vi "Send Read Geo Coding Results.vi"(7 "Message Priority (Normal)":T2=enum."Normal", 8 "error in (no error)":errorcluster, 10 "Geo Code Results":T1(array[cluster]), 11 "Message Enqueuer":refnum<class "Message Enqueuer.lvclass">) -> (0 "error out":errorcluster, 3 "Message Enqueuer out":refnum<class "Message Enqueuer.lvclass">)   [LabVIEW 2025, in "UI.lvlib" / "Read Geo Coding Results Msg.lvclass"]
doc: "This VI sends the message to an actor."
uses:
  Read Geo Coding Results Msg.lvclass
  <vilib>/ActorFramework/Message Enqueuer/Message Enqueuer.lvclass
  <vilib>/ActorFramework/Message Enqueuer/Message Priority.ctl
  C:/Program Files (x86)/National Instruments/LabVIEW 2025/vi.lib/ActorFramework/Message/Message.lvclass
  Read Geo Coding Results Msg.lvclass/Read Geo Coding Results Msg.ctl
  <vilib>/ActorFramework/Message Enqueuer/Message Enqueuer.lvclass/Message Enqueuer.ctl
  <vilib>/ActorFramework/Message Priority Queue/Priority Enqueue.vi
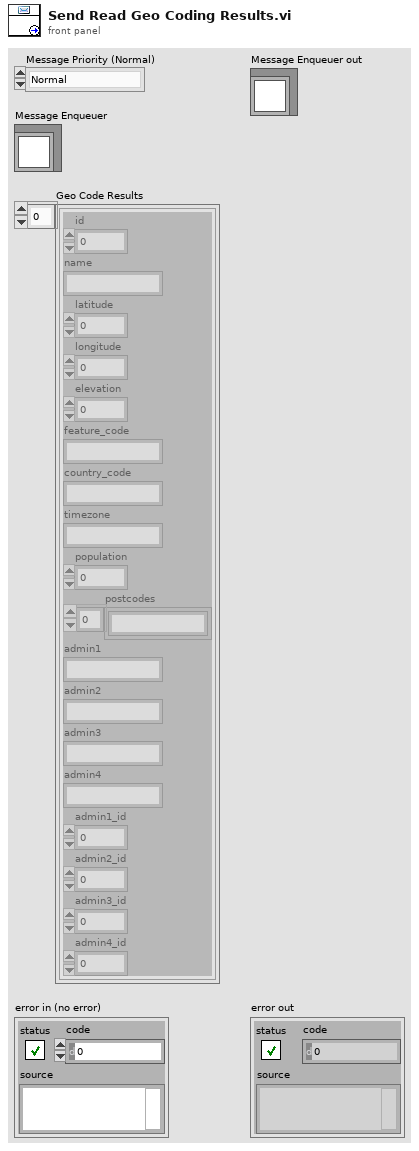
[diagram p1: front panel]
types:
  T1 = cluster{"id":i32, "name":string, "latitude":dbl, "longitude":dbl, "elevation":dbl, "feature_code":string, "country_code":string, "timezone":string, "population":i32, "postcodes":string[], "admin1":string, "admin2":string, "admin3":string, "admin4":string, "admin1_id":i32, "admin2_id":i32, "admin3_id":i32, "admin4_id":i32}[]
  T2 = typedef "Actor Framework.lvlib/Message Enqueuer.lvclass/Message Priority.ctl" = enum16{"Low", "Normal", "High"}
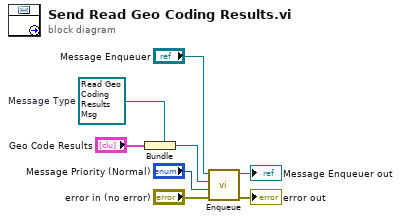
[diagram p0: block diagram]
diagram:
  w2 = refnum<class "Read Geo Coding Results Msg.lvclass"> refnum  # Message Type
  n1 = Bundle(cluster=w2, "Geo Code Results") -> (w3:refnum<class "Read Geo Coding Results Msg.lvclass">)
  n2 = call <vilib>:"Enqueue.vi"("error in (no error)"="error in (no error)", "Message Priority (Normal)"="Message Priority (Normal)", "Message"=w3, "Message Enqueuer in"="Message Enqueuer") -> ("error out"=→"error out":errorcluster, "Message Enqueuer out"=→"Message Enqueuer out":refnum<class "Message Enqueuer.lvclass">)  [unwired: 6 in]
